vi "Write Name.vi"(8 "error in (no error)":errorcluster, 10 "Name":string, 11 "Generic Driver in":refnum<class "Generic Driver.lvclass">) -> (0 "error out":errorcluster, 3 "Generic Driver out":refnum<class "Generic Driver.lvclass">)   [LabVIEW 2020, in "OOP.lvlib" / "Generic Driver.lvclass"]
uses:
  Generic Driver.lvclass
  Generic Driver.lvclass/Generic Driver.ctl
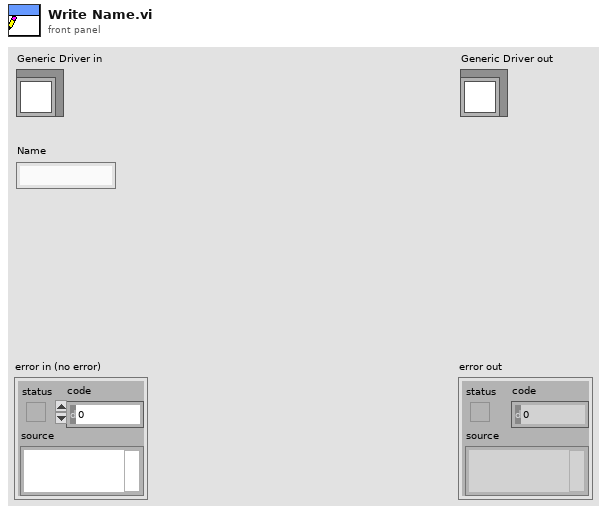
[diagram p1: front panel]
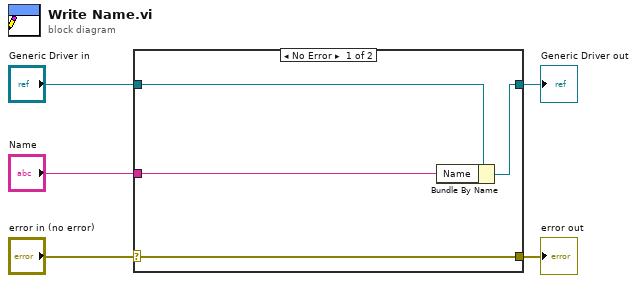
[diagram p0: block diagram]
diagram:
  n1 = case shown="No Error" "error in (no error)" {
    selector: "error in (no error)" -> [w9 w10]
    tunnel: [w9 w10] -> w4
    tunnel: [w7 w11] -> w2
    tunnel: "Generic Driver in" -> [w8 w11]
    tunnel: "Name" -> [w6 _]
    frame No Error {
      n2 = Bundle By Name(cluster=w8, "Name"=w6) -> (w7:refnum<class "Generic Driver.lvclass">)
    }
    frame Error {
    }
  }
  "error out" <- w4
  "Generic Driver out" <- w2
